vi "Export CSV.vi"(8 "error in (no error)":errorcluster, 11 "Controller in":refnum<class "Controller.lvclass">) -> (0 "error out":errorcluster, 3 "Controller out":refnum<class "Controller.lvclass">)   [LabVIEW 2013, in "SET Project Editor.lvlib" / "Controller.lvclass"]
uses:
  Controller.lvclass
  Controller.lvclass/Controller.ctl
  SET Project Data/Project Data Class/Project Data.lvclass
  SET Project Data/Resource Data Class/Resource Data.lvclass
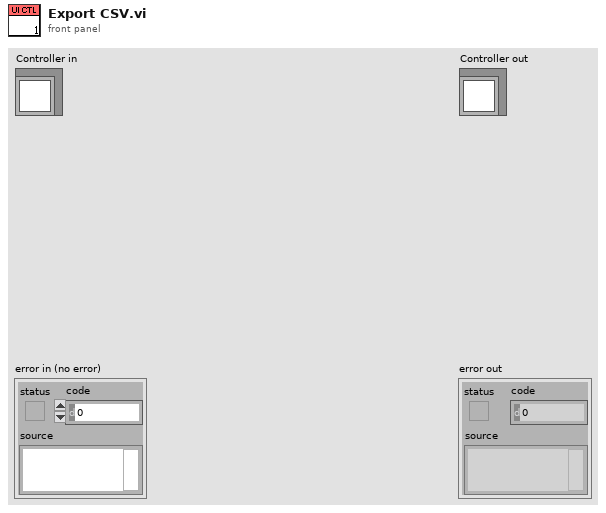
[diagram p1: front panel]
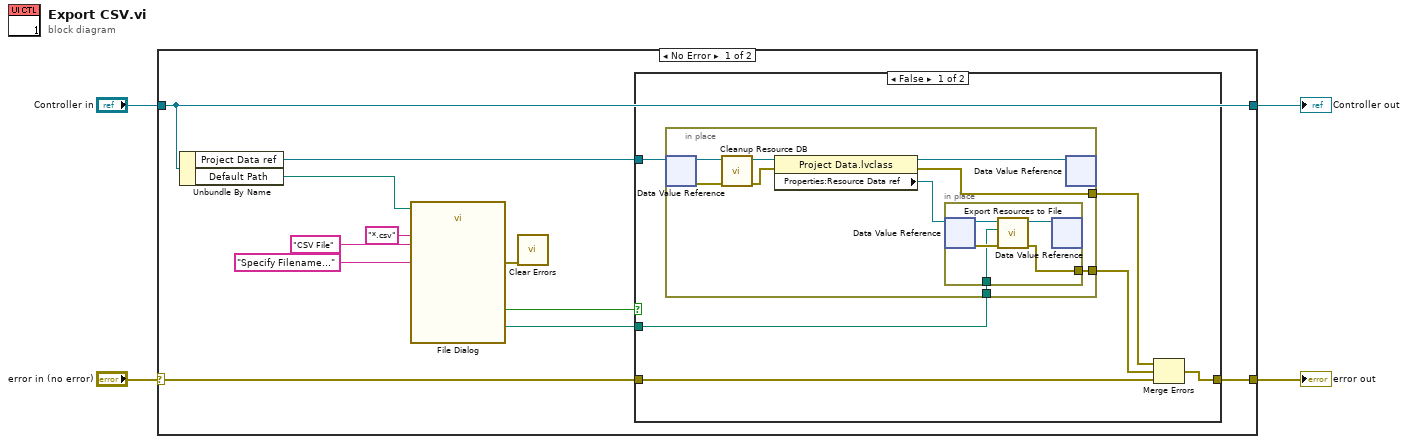
[diagram p0: block diagram]
diagram:
  n1 = case shown="No Error" "error in (no error)" {
    selector: "error in (no error)" -> [w14 w38]
    tunnel: [w13 w38] -> w3
    tunnel: [w5 w37] -> w1
    tunnel: "Controller in" -> [w5 w37]
    frame No Error {
      n2 = Unbundle By Name(w5) -> ("Project Data ref"=w15:refnum<data-value>, "Default Path"=w7:path)
      n3 = call "File Dialog"("start path"=w7, "prompt"="Specify Filename...", "pattern (all files)"="*.csv", "pattern label"="CSV File") -> ("selected path"=w8:path, "cancelled"=w6:bool, "error out"=w11:errorcluster)  [unwired: 8 in, 1 out]
      n4 = call <vilib>:"Clear Errors.vi"("error in (no error)"=w11) -> ()  [unwired: 6 in, 1 out]
      n5 = case shown="False" w6 {
        tunnel: w15 -> [w21 _]
        tunnel: w14 -> [w18 w36]
        tunnel: [w17 w36] -> w13
        tunnel: w8 -> [w16 _]
        frame False {
          n6 = in-place {
            in-place-border: [w24] -> w19
            in-place-border: [w23] -> w20
            in-place-border: w16 -> [w22]
            n7 = in-place-dvr #1(w21) -> (w29:refnum<class "Project Data.lvclass">, w28:errorcluster)
            n8 = call-dynamic "Cleanup Resource DB.vi"("error in (no error)"=w28, "ProjectData in"=w29) -> ("error out"=w26:errorcluster, "ProjectData out"=w27:refnum<class "Project Data.lvclass">)  [unwired: 8 in]
            n9 = property class="Project Data.lvclass"(reference=w27, error in=w26) -> (reference out=w25:refnum<class "Project Data.lvclass">, error out=w23:errorcluster, "Properties:Resource Data ref"=w30:refnum<data-value>)
            n10 = in-place {
              in-place-border: [w32] -> w24
              in-place-border: w22 -> [w31]
              n11 = in-place-dvr #2(w30) -> (w35:refnum<class "Resource Data.lvclass">, w33:errorcluster)
              n12 = call "Export Resources to File.vi"("error in (no error)"=w33, "File Path"=w31, "LangFile.lvclass in"=w35) -> ("error out"=w32:errorcluster, "LangFile.lvclass out"=w34:refnum<class "Resource Data.lvclass">)  [unwired: 7 in]
              n13 = in-place-dvr #2(w34) -> ()  [unwired: 2 out]
            }
            n14 = in-place-dvr #1(w25) -> ()  [unwired: 2 out]
          }
          n15 = Merge Errors(w20, w19, w18) -> (w17:errorcluster)
        }
        frame True {
        }
      }
    }
    frame Error {
    }
  }
  "error out" <- w3
  "Controller out" <- w1
